vi "Save System and Error Files.vi"() -> (2 "Error Save Path":string, 3 "System Save Path":string)   [LabVIEW 2011]
doc: "Saves the System and Error logs from Logger.VI to the default directory.\n\n\nVersion 1.0 - 02/13/2013\n\nPhaeron, Inc.\nwww.phaeron.com\ninfo@phaeron.com"
uses:
  Log Type.ctl
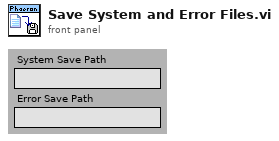
[diagram p1: front panel]
types:
  T1 = typedef "Log Type.ctl" = enum16{"System", "Data", "Error"}
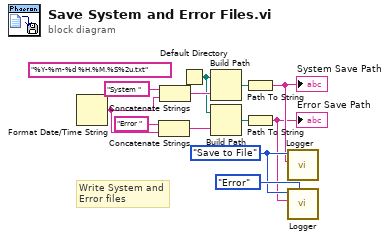
[diagram p0: block diagram]
diagram:
  (unwired) "%Y-%m-%d %H.%M.%S%2u.txt" ("time format string (%c)")
  w11 = enum16{"Init", "Read", "Append", "Save to File"}."Save to File" ("Action (Append)")
  # "Write System and\nError files"
  n1 = Format Date/Time String() -> (date/time string=w10:string)  [unwired: 3 in]
  n2 = Concatenate Strings("Error " ("time format string (%c)"), w10) -> (w9:string)
  n3 = Concatenate Strings("System " ("time format string (%c)"), w10) -> (w5:string)
  n4 = Default Directory() -> (w1:path)
  n5 = Build Path(base path=w1, name or relative path=w5) -> (appended path=w6:path)
  n6 = Build Path(base path=w1, name or relative path=w9) -> (appended path=w4:path)
  n7 = Path To String(path=w6) -> (string=w3:string)
  "System Save Path" <- w3
  n8 = Path To String(path=w4) -> (string=w2:string)
  "Error Save Path" <- w2
  n9 = call "Logger.vi"("Information"=w3, "Action (Append)"=w11) -> ()  [unwired: 6 in, 4 out]
  n10 = call "Logger.vi"("Log Type (System)"=Log_Type."Error", "Information"=w2, "Action (Append)"=w11) -> ()  [unwired: 5 in, 4 out]
